vi "Scale Potting Lines.vi"(7 "Potting Surface Type":T2, 8 "error in":errorcluster, 10 "Potting Lines":T1[](array[typedef]), 11 "Config Manager":refnum<class "Config Manager Class.lvclass">) -> (0 "error out":errorcluster, 2 "Potting Lines Scaled":T1[](array[typedef]))   [LabVIEW 2017]
uses:
  Vec3d Class/Vec3d Class.lvclass
  Type Definitions/3d Line.ctl
  Config Manager Class/Config Manager Class.lvclass
  Config Manager Class/Type Definitions/Potting Surface Type.ctl
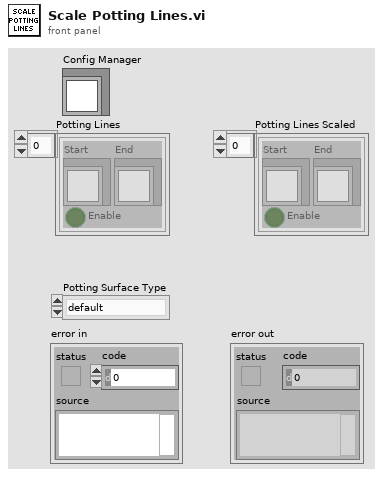
[diagram p1: front panel]
types:
  T1 = typedef "3d Line.ctl" = cluster{"Start":refnum<class "Vec3d Class.lvclass">, "End":refnum<class "Vec3d Class.lvclass">, "Enable":bool}
  T2 = typedef "Potting Surface Type.ctl" = enum16{"default", "hdi_edge_pads", "bbm_edge_pads", "address_pads"}
  T3 = typedef "FlexWorktable.lvclass/Potting Parameters.ctl" = cluster{"Curing Param A":dbl, "Curing Param B":dbl, "Speed Nominal":dbl, "Time Nominal":dbl, "Turn-on Time":dbl, "Turn-off Time":dbl, "Safe Height Offset":dbl, "Tip Height":dbl}
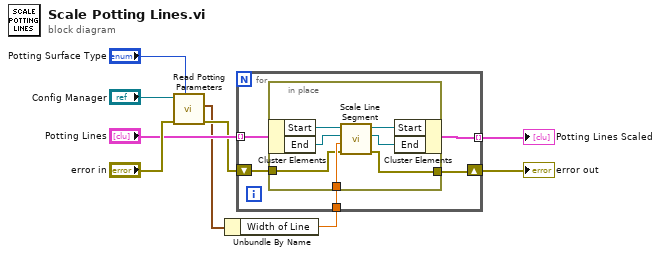
[diagram p0: block diagram]
diagram:
  n1 = call "Read Potting Parameters.vi"("Potting Surface Type"="Potting Surface Type", "error in"="error in", "Config Manager in"="Config Manager") -> ("error out"=w5:errorcluster, "Potting Parameters"=w2:T3)  [unwired: 6 in, 1 out]
  n2 = Unbundle By Name(w2) -> ("Width of Line"=w1:dbl)
  n3 = for {
    tunnel: "Potting Lines" -> [w14] mode=indexing
    shift-right: [w11] -> w4
    shift-left: w5 -> [w13]
    tunnel: [w12] -> w3 mode=indexing
    tunnel: w1 -> [w10]
    n4 = in-place {
      in-place-border: w10 -> [w19]
      in-place-border: w13 -> [w16]
      in-place-border: [w15] -> w11
      n5 = in-place-cluster #1(w14) -> ("Start"=w21:refnum<class "Vec3d Class.lvclass">, "End"=w18:refnum<class "Vec3d Class.lvclass">)
      n6 = call "Scale Line Segment.vi"("error in"=w16, "Scale Factor"=w19, "Point B in"=w18, "Point A in"=w21) -> ("error out"=w15:errorcluster, "Point B out"=w17:refnum<class "Vec3d Class.lvclass">, "Point A out"=w20:refnum<class "Vec3d Class.lvclass">)  [unwired: 5 in]
      n7 = in-place-cluster #1("Start"=w20, "End"=w17) -> (w12:T1)
    }
  }
  "error out" <- w4
  "Potting Lines Scaled" <- w3
